vi "Manual Assembly old.vi"() -> ()   [LabVIEW 2018]
uses:
  Classes/Assembly/Assembly Run.lvclass
  Classes/Controller/Controller.lvclass
  Classes/Workspace/Fixture Enum.ctl
  Classes/Workspace/Fixture.lvclass
  Classes/Routine/Routine Enum.ctl
  Classes/Routine/Routine.lvclass
panel:
  in  "Update":bool
  in  "Stage":i32(listbox)=-1
  in  "Routine":T1=enum."Dispense on Plate"
  in  "Stop":bool
  in  "Remove":bool
  in  "Add":bool
  in  "Go":bool
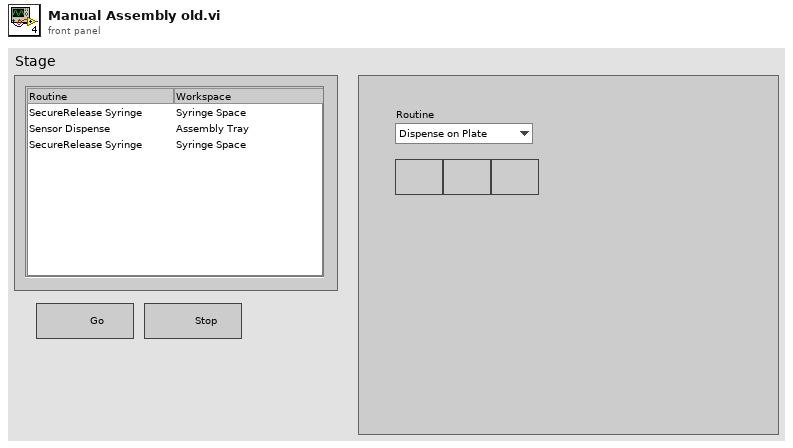
[diagram p1: front panel]
types:
  T1 = typedef "Routine.lvclass/Routine Enum.ctl" = enum16{"Primary Pick Up", "Pick Up All", "Put Down Secondary", "Put Down All", "Release Syringe", "Secondary Pick Up", "Secure Syringe", "Dispense on Plate", "Dispense on Kapton", "Dispense on Sensor"}
  T2 = typedef "Fixture.lvclass/Fixture Enum.ctl" = enum16{"Assembly Tray", "Syringe Space", "Component", "Pick Up Tool", "Current Position"}
  T3 = typedef "Controller.lvclass/Controllers.ctl" = cluster{"I-O.lvclass":refnum<class "I-O.lvclass">, "Gantry":refnum<k24>, "Dispenser":refnum<visa-resource-name>}
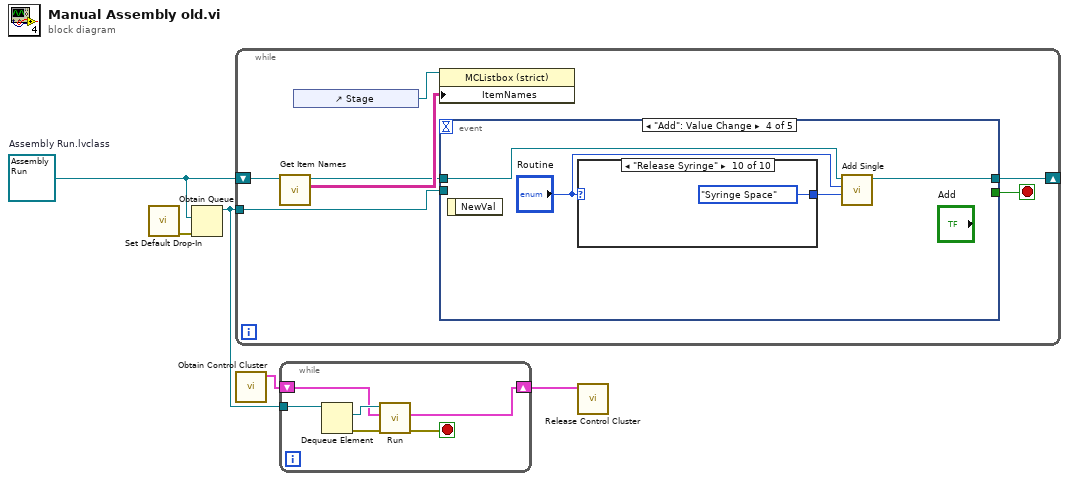
[diagram p0: block diagram]
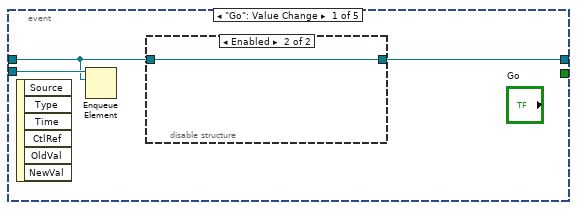
[diagram p2: hidden frame]
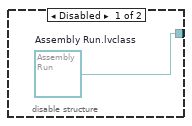
[diagram p3: hidden frame]
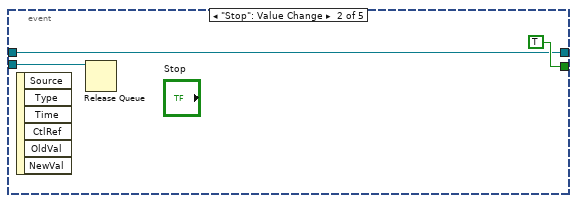
[diagram p4: hidden frame]
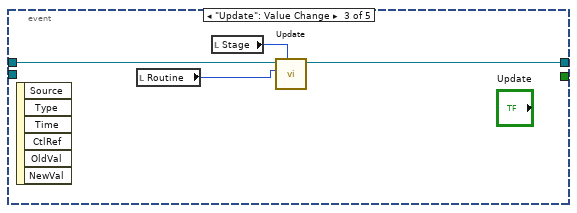
[diagram p5: hidden frame]
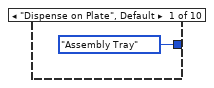
[diagram p6: hidden frame]
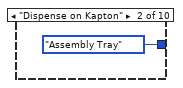
[diagram p7: hidden frame]
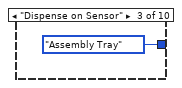
[diagram p8: hidden frame]
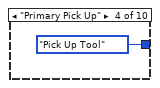
[diagram p9: hidden frame]
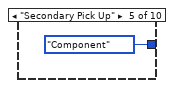
[diagram p10: hidden frame]
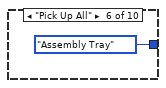
[diagram p11: hidden frame]
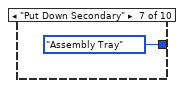
[diagram p12: hidden frame]
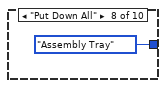
[diagram p13: hidden frame]
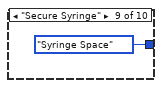
[diagram p14: hidden frame]
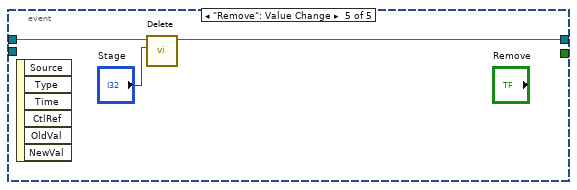
[diagram p15: hidden frame]
diagram:
  w2 = refnum<class "Assembly Run.lvclass"> refnum  # Assembly Run.lvclass
  n1 = call "Set Default Drop-In.vi"() -> ("error out"=w3:errorcluster)  [unwired: 11 in]
  n2 = Obtain Queue(element data type=w2, error in (no error)=w3) -> (queue out=w5:refnum<queue>)  [unwired: 3 in, 2 out]
  n3 = while {
    shift-right: [w6] -> _
    shift-left: w2 -> [w8]
    tunnel: w5 -> [w11]
    stop <- w12 stop-if-true
    n4 = call "Get Item Names.vi"("Assembly Run in"=w8) -> ("Item names"=w10:string[][], "Assembly Run out"=w7:refnum<class "Assembly Run.lvclass">)  [unwired: 8 in, 1 out]
    n5 = control-ref of="Stage"() -> (w9:refnum<vi>)
    n6 = property class="MCListbox (strict)"(reference=w9, "ItemNames"=w10) -> ()  [unwired: 1 in, 2 out]
    n7 = event shown="[3] \"Add\": Value Change" {
      selector: _ -> [_ _ _ _ _]
      dyn-events: _ -> [_ _ _ _ _]
      timeout: _ -> [_ _ _ _ _]
      tunnel: [_ TRUE _ _ _] -> w12
      tunnel: w7 -> [w13 w19 w24 w28 w41]
      tunnel: [w14 w19 w23 w27 w40] -> w6
      tunnel: w11 -> [w15 w18 _ _ _]
      event "Go": Value Change {
        n8 = event-data() -> ()  [unwired: 1 in, 6 out]
        n9 = Enqueue Element(queue=w15, element=w13) -> ()  [unwired: 2 in, 3 out]
        n10 = disable-structure shown="Enabled" {
          disable-tunnel: [w16 w17] -> w14
          disable-tunnel: w13 -> [_ w17]
          frame Disabled {
            w16 = refnum<class "Assembly Run.lvclass"> refnum  # Assembly Run.lvclass
          }
          frame Enabled {
          }
        }
      }
      event "Stop": Value Change {
        n11 = event-data() -> ()  [unwired: 1 in, 6 out]
        n12 = Release Queue(queue=w18) -> ()  [unwired: 2 in, 3 out]
      }
      event "Update": Value Change {
        n13 = event-data() -> ()  [unwired: 1 in, 6 out]
        n14 = local read "Routine"() -> (w22:T1)
        n15 = local read "Stage"() -> (w21:i32)
        n16 = call "Update.vi"("Row"=w21, "Routine"=w22, "Assembly Run in"=w24) -> ("Assembly Run out"=w23:refnum<class "Assembly Run.lvclass">)  [unwired: 7 in, 1 out]
      }
      event "Add": Value Change {
        n17 = event-data() -> ()  [unwired: 1 in, 1 out]
        n18 = case shown="\"Release Syringe\"" "Routine" {
          tunnel: [Fixture_Enum."Assembly Tray" ("Fixture") Fixture_Enum."Assembly Tray" ("Fixture") Fixture_Enum."Assembly Tray" ("Fixture") Fixture_Enum."Pick Up Tool" ("Fixture") Fixture_Enum."Component" ("Fixture") Fixture_Enum."Assembly Tray" ("Fixture") Fixture_Enum."Assembly Tray" ("Fixture") Fixture_Enum."Assembly Tray" ("Fixture") Fixture_Enum."Syringe Space" ("Fixture") Fixture_Enum."Syringe Space" ("Fixture")] -> w25
          frame "Dispense on Plate", Default {
          }
          frame "Dispense on Kapton" {
          }
          frame "Dispense on Sensor" {
          }
          frame "Primary Pick Up" {
          }
          frame "Secondary Pick Up" {
          }
          frame "Pick Up All" {
          }
          frame "Put Down Secondary" {
          }
          frame "Put Down All" {
          }
          frame "Secure Syringe" {
          }
          frame "Release Syringe" {
          }
        }
        n19 = call-dynamic "Add Single.vi"("Fixture"=w25, "Routine"="Routine", "UI in"=w28) -> ("UI out"=w27:refnum<class "Assembly Run.lvclass">)  [unwired: 6 in, 1 out]
      }
      event "Remove": Value Change {
        n20 = event-data() -> ()  [unwired: 1 in, 6 out]
        n21 = call "Delete.vi"("Index"="Stage", "Assembly In"=w41) -> ("Assembly Out"=w40:refnum<class "Assembly Run.lvclass">)  [unwired: 8 in, 1 out]
      }
    }
  }
  n22 = call "Obtain Control Cluster.vi"() -> ("Control Out"=w1:T3)  [unwired: 11 in]
  n23 = while {
    tunnel: w5 -> [w47]
    shift-right: [w42] -> w4
    shift-left: w1 -> [w43]
    stop <- w44 stop-if-true
    n24 = Dequeue Element(queue=w47) -> (element=w46:refnum<class "Assembly Run.lvclass">, error out=w45:errorcluster)  [unwired: 2 in, 2 out]
    n25 = call-dynamic "Run.vi"("error in (no error)"=w45, "Control In"=w43, "Assembly In"=w46) -> ("error out"=w44:errorcluster, "Control Out"=w42:T3)  [unwired: 6 in, 1 out]
  }
  n26 = call "Release Control Cluster.vi"("output cluster"=w4) -> ()  [unwired: 11 in]
